vi "Get Central Message Handler.vi"(8 "Error In":errorcluster, 11 "Dashboard In":refnum<class "Dashboard.lvclass">) -> (0 "Error Out":errorcluster, 2 "Central Message Handler":refnum<class "Central Message Handler.lvclass">, 3 "Dashboard Out":refnum<class "Dashboard.lvclass">)   [LabVIEW 2019, in "Dashboard.lvclass"]
uses:
  Dashboard.lvclass
  Central Message Handler/Central Message Handler.lvclass
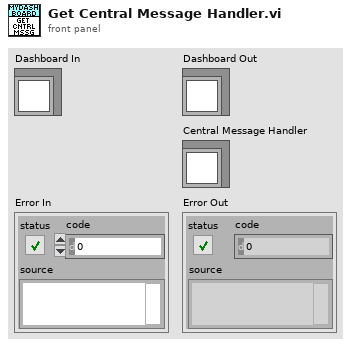
[diagram p1: front panel]
types:
  T1 = typedef "Dashboard.lvclass/Data.ctl" = cluster{"Central Message Handler":refnum<class "Central Message Handler.lvclass">, "Display":refnum<class "Display.lvclass">, "FPGA Reference":T2, "Open Weather Session":refnum<class "Open Weather Session.lvclass">, "Processes":T3}
  T2 = typedef "Dashboard.lvclass/FPGA Reference.ctl" = refnum<k20>
  T3 = typedef "Dashboard.lvclass/Processes.ctl" = cluster{"Display Manager":refnum<class "Display Manager.lvclass">, "Audio Analyzer":refnum<class "Audio Analyzer.lvclass">, "Draw Frame":refnum<class "Draw Frame.lvclass">, "Error Handling":refnum<class "Error Handling.lvclass">, "Sequencer":refnum<class "Sequencer.lvclass">}
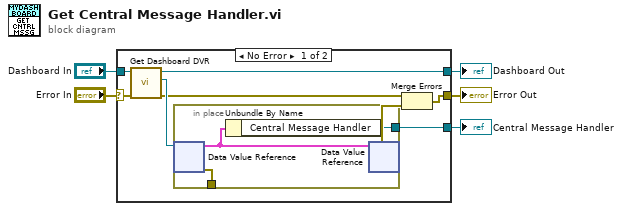
[diagram p0: block diagram]
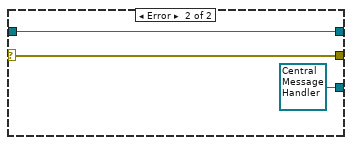
[diagram p2: hidden frame]
diagram:
  n1 = case shown="No Error" "Error In" {
    selector: "Error In" -> [w10 w18]
    tunnel: [w12 w18] -> w2
    tunnel: [w9 w19] -> w4
    tunnel: "Dashboard In" -> [w11 w19]
    tunnel: [w6 refnum<class "Central Message Handler.lvclass"> refnum ("Central Message Handler")] -> w1
    frame No Error {
      n2 = call "Get Dashboard DVR.vi"("Error In"=w10, "Dashboard In"=w11) -> ("Error Out"=w7:errorcluster, "DVR"=w8:refnum<data-value>, "Dashboard Out"=w9:refnum<class "Dashboard.lvclass">)  [unwired: 7 in]
      n3 = in-place {
        in-place-border: [w14] -> w6
        in-place-border: [w16] -> _
        n4 = in-place-dvr #1(w8) -> (w15:T1, w16:errorcluster)
        n5 = Unbundle By Name(w15) -> ("Central Message Handler"=w14:refnum<class "Central Message Handler.lvclass">)
        n6 = in-place-dvr #1(w15) -> (w13:errorcluster)  [unwired: 1 out]
      }
      n7 = Merge Errors(w7, w13) -> (w12:errorcluster)
    }
    frame Error {
    }
  }
  "Dashboard Out" <- w4
  "Error Out" <- w2
  "Central Message Handler" <- w1
